vi "Read Variable Reluctance all channels.vi"() -> ()   [LabVIEW 8.6]
uses:
  <libdir>/resource/objmgr/UeiDaq.rc
  <vilib>/UeiDaq/UeiDaqConfigureTimingForSimpleIO.vi
panel:
  in  "Channel configuration":cluster{"ZC Mode":i32, "APT Mode":i32}[](array[cluster]) {"APT Mode" items=["Chip", "Logic", "Fixed", "TTL"]; "ZC Mode" items=["Chip", "Logic", "Fixed"]}
  out "open circuit":bool[](array[boolean])
  in  "channel":i32
  out "input freq":dbl
  in  "channel":i32
  out "Number of FIFO values read":i32[](array[numeric])
  out "FIFO Values":u32[][](array[numeric])
  in  "Number of values":i32
  in  "Channel":i32
  out "Values":T1(array[cluster])
  in  "ADC Rate ( hz )":dbl
  out "Number of ADC values read":i32
  out "ADC data":dbl[][](graph)
  out "Position":u32(graph)
  in  "Channel settings":T2(array[cluster]) {"ADC moving avg" items=["off", "on (8x)"]; "Mode" items=["Decoder", "Timed", "N Pulses", "Z Pulse"]}
  out "Serial Number":string
  out "Name":string
  in  "Device and channels":string
  out "Total values acquired":u32
  in  "stop":bool
  # "VR-608 Variable Reluctance input - all channels"
  # "This example displays the functionality of the VR-608 to measure in either timed, n-pulse, z-pulse or\ndecoder modes while setting the number of teeth and z-tooth size. The velocity, position, teeth count, and\ntimestamp are displayed."
  # "Set ZC thresh (V) and APC thresh(V) in fixed APT and ZC modes"
  # "Z tooth size: missing teeth (-1 to -3) or long teeth (1 to 3)"
  # "normalize velocity to input frequency"
  # "0/1"
  # "0"
  # "Results"
  # "0"
  # "1"
  # "2"
  # "3"
  # "4"
  # "5"
  # "6"
  # "7"
  # "2/3"
  # "1"
  # "4/5"
  # "2"
  # "6/7"
  # "3"
  # "4"
  # "ZC: Zero-crossing mode"
  # "APT: adaptive peak threshold \nmode"
  # "5"
  # "APT mode sets the peak \nthreshold to 1/3 of the peak \ninput voltage"
  # "6"
  # "7"
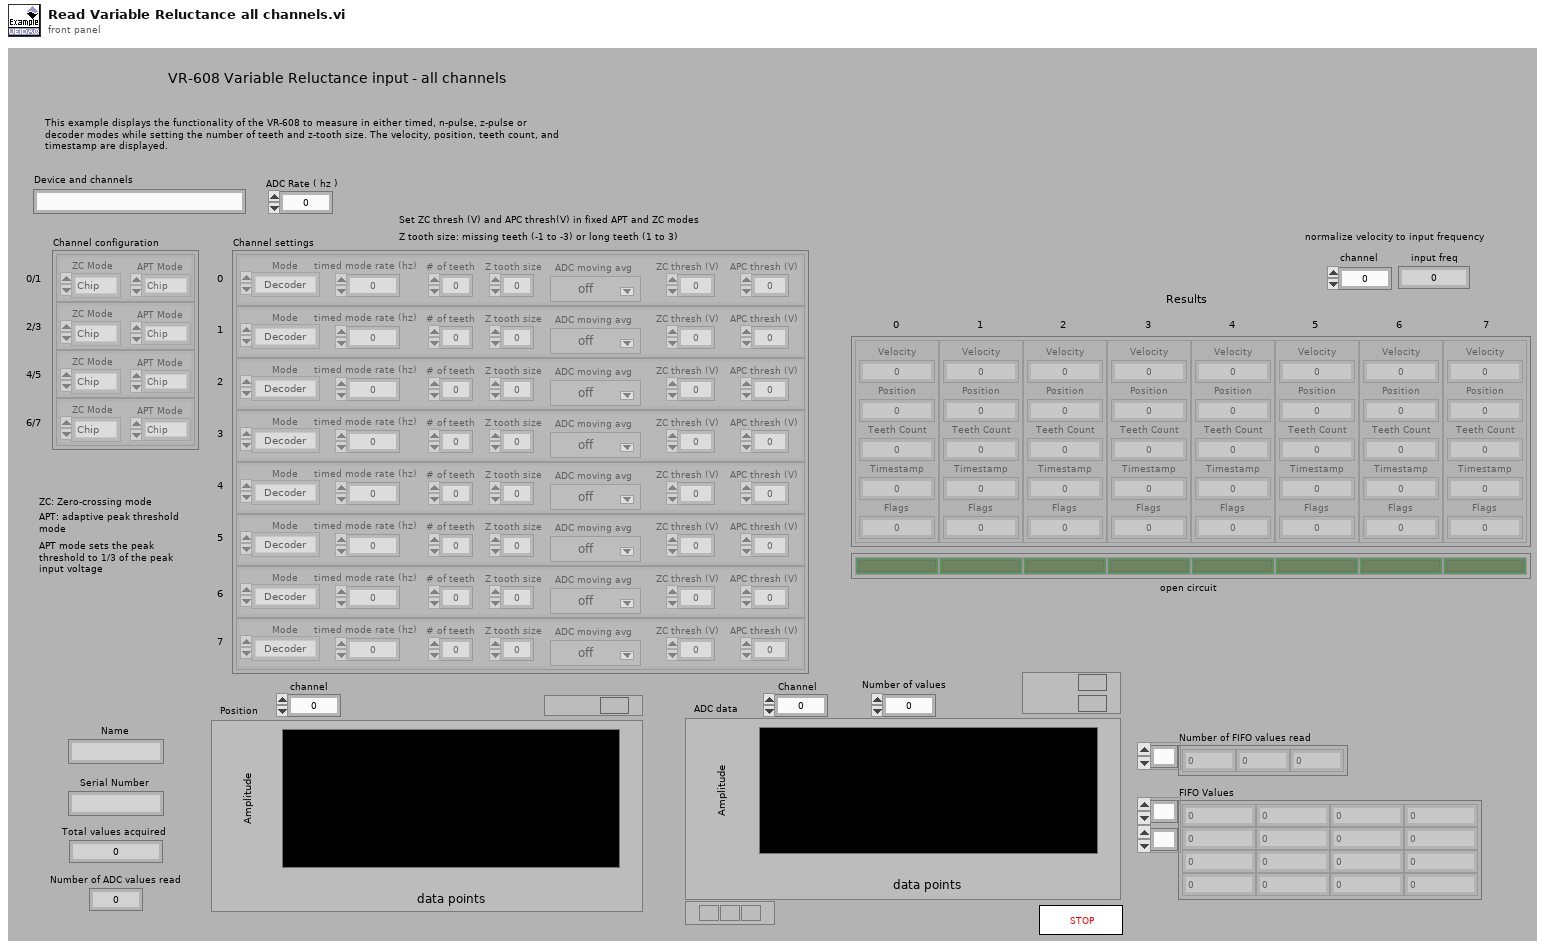
[diagram p1: front panel]
types:
  T1 = cluster{"Velocity":dbl, "Position":u32, "Teeth Count":u32, "Timestamp":u32, "Flags":u32}[]
  T2 = cluster{"Mode":i32, "timed mode rate (hz)":dbl, "# of teeth":i32, "Z tooth size":i32, "ADC moving avg":i32, "ZC thresh (V)":dbl, "APC thresh (V)":dbl}[]
  T3 = cluster{"Velocity":dbl, "Position":u32, "Teeth Count":u32, "Timestamp":u32, "Flags":u32}
  T4 = cluster{"Mode":i32, "timed mode rate (hz)":dbl, "# of teeth":i32, "Z tooth size":i32, "ADC moving avg":i32, "ZC thresh (V)":dbl, "APC thresh (V)":dbl}
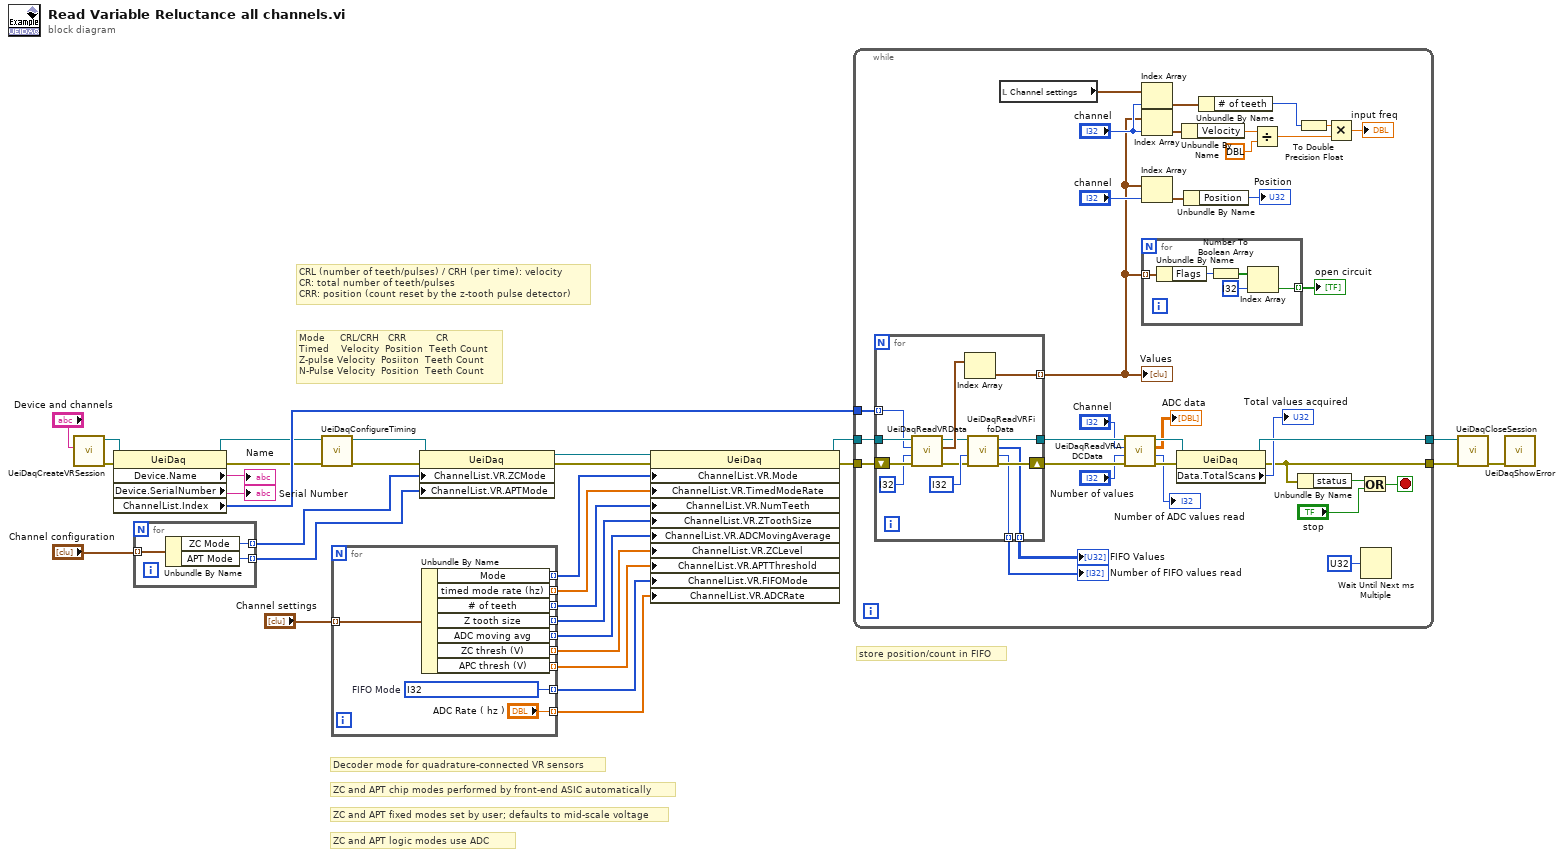
[diagram p0: block diagram]
diagram:
  # "Mode     CRL/CRH   CRR          CR\nTimed    Velocity  Position  Teeth Count\nZ-pulse Velocity  Posiiton  Teeth Count\nN-Pulse Velocity  Position  Teeth Count"
  # "CRL (number of teeth/pulses) / CRH (per time): velocity\nCR: total number of teeth/pulses\nCRR: position (count reset by the z-tooth pulse detector)"
  # "store position/count in FIFO"
  # "ZC and APT fixed modes set by user; defaults to mid-scale voltage"
  # "ZC and APT chip modes performed by front-end ASIC automatically"
  # "Decoder mode for quadrature-connected VR sensors"
  # "ZC and APT logic modes use ADC"
  n1 = call <vilib>:"UeiDaqCreateVRSession.vi"("Resource"="Device and channels") -> ("error out"=w20:errorcluster, "UeiDaq Refnum Out"=w21:refnum<k20>)  [unwired: 3 in, 6 out]
  n2 = property class="UeiDaq"(reference=w21, error in=w20) -> (reference out=w18:refnum<k20>, error out=w19:errorcluster, "Device.Name"=→"Name":string, "Device.SerialNumber"=→"Serial Number":string, "ChannelList.Index"=w23:i32[])
  n3 = for {
    tunnel: "Channel configuration" -> [w33] mode=indexing
    tunnel: [w32] -> w6 mode=indexing
    tunnel: [w31] -> w7 mode=indexing
    n4 = Unbundle By Name(w33) -> ("ZC Mode"=w32:i32, "APT Mode"=w31:i32)
  }
  n5 = call-poly <vilib>:"UeiDaqConfigureTiming.vi"("error in (no error)"=w19, "UeiDaq Refnum In"=w18) -> ("error out"=w12:errorcluster, "UeiDaq Refnum Out"=w14:refnum<k20>)  [unwired: 1 in, 7 out]
  n6 = for {
    tunnel: "Channel settings" -> [w43] mode=indexing
    tunnel: [w42] -> w8 mode=indexing
    tunnel: [w41] -> w1 mode=indexing
    tunnel: [w40] -> w16 mode=indexing
    tunnel: [w39] -> w15 mode=indexing
    tunnel: [w38] -> w2 mode=indexing
    tunnel: [w37] -> w3 mode=indexing
    tunnel: ["ADC Rate ( hz )"] -> w9 mode=indexing
    tunnel: [w35] -> w5 mode=indexing
    tunnel: [w34] -> w4 mode=indexing
    w35 = i32 ? items=["Disabled", "Position", "PositionAndTimestamp"]  # FIFO Mode
    n7 = Unbundle By Name(w43) -> ("Mode"=w42:i32, "timed mode rate (hz)"=w41:dbl, "# of teeth"=w40:i32, "Z tooth size"=w39:i32, "ADC moving avg"=w38:i32, "ZC thresh (V)"=w37:dbl, "APC thresh (V)"=w34:dbl)
  }
  n8 = property class="UeiDaq"(reference=w14, error in=w12, "ChannelList.VR.ZCMode"=w6, "ChannelList.VR.APTMode"=w7) -> (reference out=w13:refnum<k20>, error out=w11:errorcluster)
  n9 = property class="UeiDaq"(reference=w13, error in=w11, "ChannelList.VR.Mode"=w8, "ChannelList.VR.TimedModeRate"=w1, "ChannelList.VR.NumTeeth"=w16, "ChannelList.VR.ZToothSize"=w15, "ChannelList.VR.ADCMovingAverage"=w2, "ChannelList.VR.ZCLevel"=w3, "ChannelList.VR.APTThreshold"=w4, "ChannelList.VR.FIFOMode"=w5, "ChannelList.VR.ADCRate"=w9) -> (reference out=w27:refnum<k20>, error out=w28:errorcluster)
  n10 = while {
    tunnel: w27 -> [w77]
    tunnel: w28 -> [w78]
    tunnel: [w74] -> w26
    tunnel: [w76] -> w25
    tunnel: w23 -> [w69]
    stop <- w71 stop-if-true
    n11 = for {
      tunnel: w77 -> [w95]
      tunnel: [w86] -> w66
      shift-right: [w88] -> w63
      shift-left: w78 -> [w96]
      tunnel: w69 -> [w91] mode=indexing
      tunnel: [w92] -> w45 mode=indexing
      tunnel: [w85] -> w58 mode=indexing
      tunnel: [w84] -> w59 mode=indexing
      n12 = call <vilib>:"UeiDaqReadVRData.vi"("error in (no error)"=w96, "Number of values"=i32 ?, "Channel"=w91, "UeiDaq Refnum In"=w95) -> ("error out"=w89:errorcluster, "Values"=w93:T1, "UeiDaq Refnum Out"=w87:refnum<k20>)  [unwired: 5 out]
      n13 = Index Array(array=w93) -> (element=w92:T3)  [unwired: 1 in]
      n14 = call <vilib>:"UeiDaqReadVRFifoData.vi"("error in (no error)"=w89, "Number of values"=i32 ?, "UeiDaq Refnum In"=w87) -> ("error out"=w88:errorcluster, "Number of values read"=w84:i32, "FIFO Values"=w85:u32[], "UeiDaq Refnum Out"=w86:refnum<k20>)  [unwired: 1 in, 4 out]
    }
    "Values" <- w45
    "FIFO Values" <- w58
    "Number of FIFO values read" <- w59
    n15 = local read "Channel settings"() -> (w53:T2)
    n16 = call <vilib>:"UeiDaqReadVRADCData.vi"("error in (no error)"=w63, "Number of values"="Number of values", "Channel"="Channel", "UeiDaq Refnum In"=w66) -> ("error out"=w64:errorcluster, "Number of values read"=→"Number of ADC values read":i32, "ADC Values"=→"ADC data":dbl[][], "UeiDaq Refnum Out"=w65:refnum<k20>)  [unwired: 4 out]
    n17 = Index Array(array=w53, index="channel") -> (element=w51:T4)
    n18 = Index Array(array=w45, index="channel") -> (element=w52:T3)
    n19 = Index Array(array=w45, index="channel") -> (element=w68:T3)
    n20 = for {
      tunnel: w45 -> [w83] mode=indexing
      tunnel: [w80] -> w44 mode=indexing
      n21 = Unbundle By Name(w83) -> ("Flags"=w82:u32)
      n22 = Number To Boolean Array(number=w82) -> (Boolean array=w81:bool[])
      n23 = Index Array(array=w81, index=i32 ?) -> (element=w80:bool)
    }
    "open circuit" <- w44
    n24 = property class="UeiDaq"(reference=w65, error in=w64) -> (reference out=w76:refnum<k20>, error out=w74:errorcluster, "Data.TotalScans"=→"Total values acquired":u32)
    n25 = Unbundle By Name(w52) -> ("Velocity"=w55:dbl)
    n26 = Unbundle By Name(w68) -> ("Position"=→"Position":u32)
    n27 = Unbundle By Name(w51) -> ("# of teeth"=w49:i32)
    n28 = Divide(x=w55, y=dbl ?) -> (x/y=w50:dbl)
    n29 = Unbundle By Name(w74) -> ("status"=w72:bool)
    n30 = To Double Precision Float(number=w49) -> (double precision float=w48:dbl)
    n31 = Multiply(x=w48, y=w50) -> (x*y=→"input freq":dbl)
    n32 = Or(x=w72, y="stop") -> (x .or. y?=w71:bool)
    n33 = Wait Until Next ms Multiple(millisecond multiple=u32 ?) -> ()  [unwired: 1 out]
  }
  n34 = call <vilib>:"UeiDaqCloseSession.vi"("error in (no error)"=w26, "UeiDaq Refnum In"=w25) -> ("error out"=w30:errorcluster)  [unwired: 1 in, 8 out]
  n35 = call <vilib>:"UeiDaqShowError.vi"("error in (no error)"=w30) -> ()  [unwired: 1 in, 10 out]
